vi "PopulateArray (SubVI).vi"(9 "Array in":i32[](array[numeric]), 10 "Numeric":i32, 11 "Boolean":bool) -> (3 "Array out":i32[](array[numeric]))   [LabVIEW 2017]
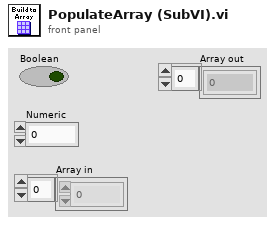
[diagram p1: front panel]
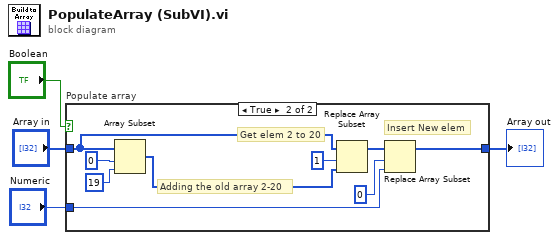
[diagram p0: block diagram]
diagram:
  n1 = case "Populate array" shown="True" "Boolean" {
    tunnel: "Array in" -> [w5 w10]
    tunnel: "Numeric" -> [_ w8]
    tunnel: [w5 w7] -> w4
    frame False {
    }
    frame True {
      # "Insert New elem"
      # "Adding the old array 2-20"
      # "Get elem 2 to 20"
      n2 = Array Subset(array=w10, index=0, length=19) -> (w12:i32[])
      n3 = Replace Array Subset(array=w10, new element=w12, index=1) -> (w6:i32[])
      n4 = Replace Array Subset(array=w6, new element=w8, index=0) -> (w7:i32[])
    }
  }
  "Array out" <- w4
